vi "hse-configuration_ReadDataDirectory.vi"(8 "error in (no error)":errorcluster, 11 "hse-configuration in":refnum<class "hse-configuration.lvclass">) -> (0 "error out":errorcluster, 2 "Data Directory":variant, 3 "hse-configuration out":refnum<class "hse-configuration.lvclass">)   [LabVIEW 2014, in "hse-configuration.lvclass"]
uses:
  hse-configuration.lvclass
  hse-configuration.lvclass/hse-configuration.ctl
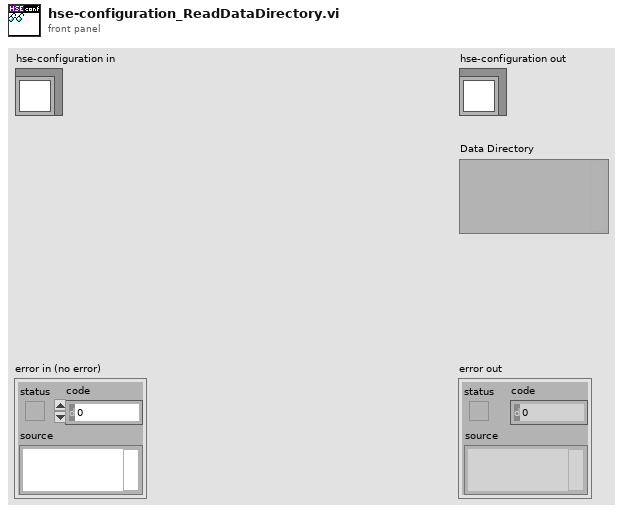
[diagram p1: front panel]
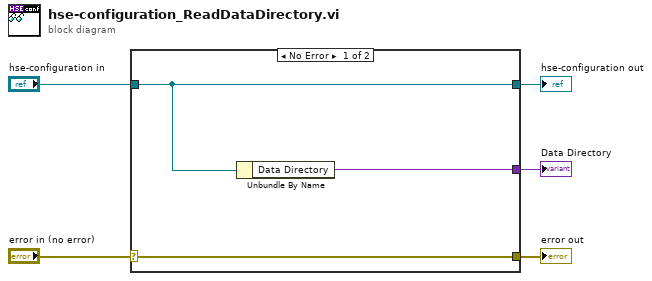
[diagram p0: block diagram]
diagram:
  n1 = case shown="No Error" "error in (no error)" {
    selector: "error in (no error)" -> [w8 w9]
    tunnel: [w8 w9] -> w4
    tunnel: [w7 w10] -> w2
    tunnel: "hse-configuration in" -> [w7 w10]
    tunnel: [w6 _] -> w1
    frame No Error {
      n2 = Unbundle By Name(w7) -> ("Data Directory"=w6:variant)
    }
    frame Error {
    }
  }
  "error out" <- w4
  "hse-configuration out" <- w2
  "Data Directory" <- w1
